vi "Write Tags.vi"(8 "error in (no error)":errorcluster, 11 "Cluster in":T1) -> (0 "error out":errorcluster, 3 "Cluster out":T1)   [LabVIEW 2019, in "Data Publishing Service.lvlib"]
uses:
  Data Publishing Service.lvlib
  Types/State Variables.ctl
  Types/INI Configuration.ctl
  <vilib>/NI VeriStand/Execution/Workspace/WorkspaceAPI.ctl
  NationalInstruments.VeriStand.ClientAPI
  <vilib>/NI VeriStand/Execution/AlarmManager/AlarmManagerAPI.ctl
  <vilib>/Skyline/Tag/Wrapper/Wrapper_class/NI Skyline Tag.lvclass
  <vilib>/NI VeriStand/Execution/Alarm/AlarmAPI.ctl
  <vilib>/Skyline/Tag/Shared/Serialize Double to String.vi
  <vilib>/NI VeriStand/Execution/Workspace/NI VeriStand - Get Multiple Channel Values.vi
  <vilib>/Skyline/Tag/Wrapper/Wrapper_class/Generate Tag Cluster 2.vi
  <vilib>/Skyline/Tag/Wrapper/Wrapper_class/Generate Tag Cluster (DBL) 2.vi
  <vilib>/Skyline/Tag/Wrapper/Wrapper_class/Multi Write 2.vi
  <vilib>/Skyline/Tag/Wrapper/Wrapper_class/Generate Tag Cluster (String) 2.vi
  <vilib>/Skyline/Configuration/Configuration_class/NI Skyline Configuration.lvclass
  <vilib>/NI VeriStand/Execution/Workspace/NI_VS Workspace ExecutionAPI.lvlib
  <vilib>/NI VeriStand/Execution/Alarm/NI_VS Alarm ExecutionAPI.lvlib
  <vilib>/NI VeriStand/Execution/AlarmManager/NI_VS AlarmManager ExecutionAPI.lvlib
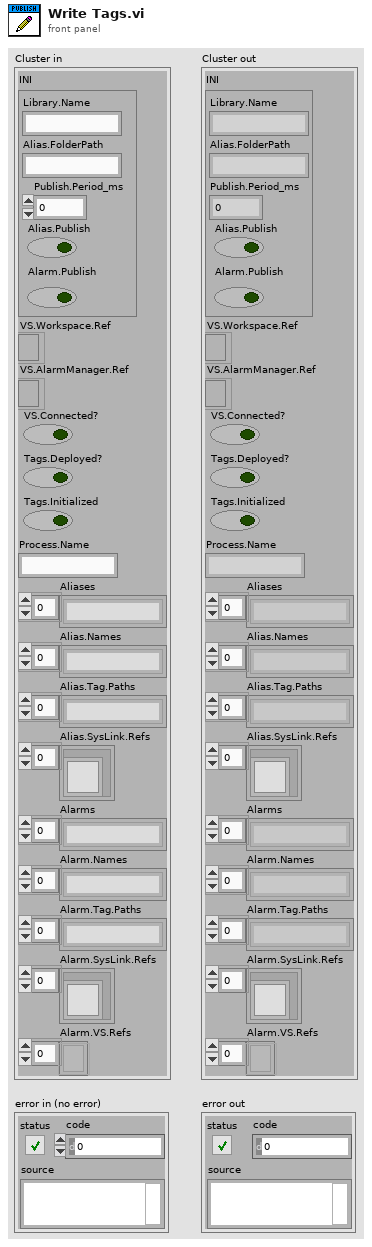
[diagram p1: front panel]
types:
  T1 = typedef "Data Publishing Service.lvlib/State Variables.ctl" = cluster{"INI":T2, "VS.Workspace.Ref":T3, "VS.AlarmManager.Ref":T4, "VS.Connected?":bool, "Tags.Deployed?":bool, "Tags.Initialized":bool, "Process.Name":string, "Aliases":string[], "Alias.Names":string[], "Alias.Tag.Paths":string[], "Alias.SysLink.Refs":refnum<class "NI Skyline Tag.lvclass">[], "Alarms":string[], "Alarm.Names":string[], "Alarm.Tag.Paths":string[], "Alarm.SysLink.Refs":refnum<class "NI Skyline Tag.lvclass">[], "Alarm.VS.Refs":T5[]}
  T2 = typedef "Data Publishing Service.lvlib/INI Configuration.ctl" = cluster{"Library.Name":string, "Alias.FolderPath":string, "Publish.Period_ms":u32, "Alias.Publish":bool, "Alarm.Publish":bool}
  T3 = typedef "NI_VS Workspace ExecutionAPI.lvlib/WorkspaceAPI.ctl" = refnum<k24>
  T4 = typedef "NI_VS AlarmManager ExecutionAPI.lvlib/AlarmManagerAPI.ctl" = refnum<k24>
  T5 = typedef "NI_VS Alarm ExecutionAPI.lvlib/AlarmAPI.ctl" = refnum<k24>
  T6 = typedef "NI_VS Alarm ExecutionAPI.lvlib/AlarmInfo.ctl" = cluster{"Watch Channel":string, "High Limit Constant":bool, "High Limit Channel":string, "High Limit":dbl, "Low Limit Constant":bool, "Low Limit Channel":string, "Low Limit":dbl, "Procedure Name":string, "Delay":dbl, "Trip Value":dbl, "Priority":enum16{"Low", "Medium", "High"}, "State":enum16{"Disabled", "Enabled", "Tripped", "Delayed Trip", "Indicate"}, "Mode":enum16{"Normal", "Indicate Only"}, "Group Number":u32, "Priority Number":u32, "Name":string, "Full Name":string}
  T7 = enum16{"Disabled", "Enabled", "Tripped", "Delayed Trip", "Indicate"}
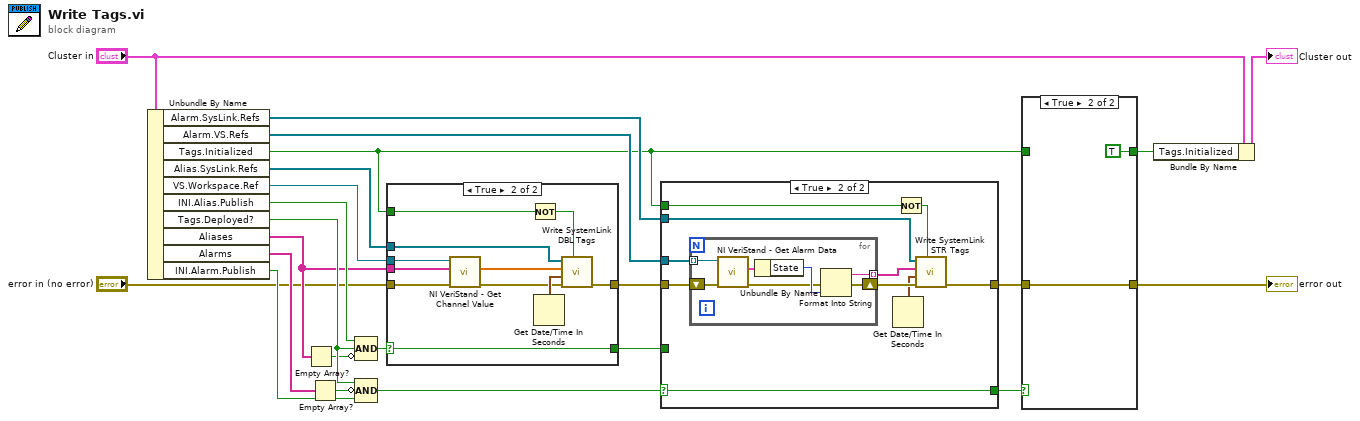
[diagram p0: block diagram]
diagram:
  n1 = Unbundle By Name("Cluster in") -> ("Alarm.SysLink.Refs"=w2:refnum<class "NI Skyline Tag.lvclass">[], "Alarm.VS.Refs"=w15:T5[], "Tags.Initialized"=w1:bool, "Alias.SysLink.Refs"=w3:refnum<class "NI Skyline Tag.lvclass">[], "VS.Workspace.Ref"=w4:T3, "INI.Alias.Publish"=w10:bool, "Tags.Deployed?"=w17:bool, "Aliases"=w9:string[], "Alarms"=w13:string[], "INI.Alarm.Publish"=w18:bool)
  n2 = Empty Array?(array=w9) -> (empty?=w8:bool)
  n3 = Empty Array?(array=w13) -> (empty?=w12:bool)
  n4 = Compound Arithmetic op=AND(w10, w17, invert w8) -> (w16:bool)
  n5 = Compound Arithmetic op=AND(w17, invert w12, w18) -> (w11:bool)
  n6 = case shown="True" w16 {
    selector: w16 -> [w24 w33]
    tunnel: [w25 w30] -> w14
    tunnel: "error in (no error)" -> [w25 w36]
    tunnel: w4 -> [_ w35]
    tunnel: w9 -> [_ w34]
    tunnel: [w24 w33] -> w22
    tunnel: w3 -> [_ w28]
    tunnel: w1 -> [_ w27]
    frame False {
    }
    frame True {
      n7 = call-poly <vilib>:"NI VeriStand - Get Channel Value.vi"("error in (no error)"=w36, "Channels"=w34, "WorkspaceManager in"=w35) -> ("error out"=w31:errorcluster, "Values"=w29:dbl[])  [unwired: 6 in, 1 out]
      n8 = Not(x=w27) -> (.not. x?=w26:bool)
      n9 = Get Date/Time In Seconds() -> (seconds since 1Jan1904=w32:timestamp)
      n10 = call "Write SystemLink DBL Tags.vi"("Force Initialize?"=w26, "error in (no error)"=w31, "timestamp"=w32, "Values"=w29, "SkyLine.Refs"=w28) -> ("error out"=w30:errorcluster)  [unwired: 6 in]
    }
  }
  n11 = case shown="True" w11 {
    selector: w11 -> [_ w46]
    tunnel: [w38 w44] -> w19
    tunnel: w14 -> [w38 w48]
    tunnel: w15 -> [_ w47]
    tunnel: w22 -> [w37 _]
    tunnel: [w37 w46] -> w23
    tunnel: w2 -> [_ w41]
    tunnel: w1 -> [_ w40]
    frame False {
    }
    frame True {
      n12 = for {
        shift-right: [w50] -> w45
        shift-left: w48 -> [w55]
        tunnel: w47 -> [w54] mode=indexing
        tunnel: [w49] -> w42 mode=indexing
        n13 = call <vilib>:"NI VeriStand - Get Alarm Data.vi"("error in (no error)"=w55, "Alarm in"=w54) -> ("error out"=w51:errorcluster, "Alarm Data"=w53:T6)  [unwired: 7 in, 1 out]
        n14 = Unbundle By Name(w53) -> ("State"=w52:T7)
        n15 = Format Into String(error in=w51, w52) -> (resulting string=w49:string, error out=w50:errorcluster)  [unwired: 2 in]
      }
      n16 = Get Date/Time In Seconds() -> (seconds since 1Jan1904=w43:timestamp)
      n17 = Not(x=w40) -> (.not. x?=w39:bool)
      n18 = call "Write SystemLink STR Tags.vi"("Force Initialize?"=w39, "error in (no error)"=w45, "timestamp"=w43, "Values"=w42, "SkyLine.Refs"=w41) -> ("error out"=w44:errorcluster)  [unwired: 6 in]
    }
  }
  n19 = case shown="True" w23 {
    tunnel: w1 -> [w56 _]
    tunnel: w19 -> [w57 w58]
    tunnel: [w57 w58] -> w20
    tunnel: [w56 TRUE ("Tags.Initialized")] -> w21
    frame False {
    }
    frame True {
    }
  }
  "error out" <- w20
  n20 = Bundle By Name(cluster="Cluster in", "Tags.Initialized"=w21) -> (→"Cluster out":T1)
